vi "Update Sampling Rate.vi"(8 "error in (no error)":errorcluster, 10 "Timing Parameter":T1={"rate"=1000.0, "samples per channel"=1000, "sample mode"=10123} {"sample mode" items=["Finite Samples"=10178, "Continuous Samples"=10123, "Hardware Timed Single Point"=12522]; "rate" format="%0.2f"}, 11 "Abstract in":refnum<class "Abstract.lvclass">) -> (0 "error out":errorcluster, 3 "Abstract out":refnum<class "Abstract.lvclass">)   [LabVIEW 2016, in "DAQ Hardware.lvlib" / "Abstract.lvclass"]
uses:
  Abstract.lvclass
  Timing AI DAQ Setting.ctl
  DAQ Hardware.lvlib
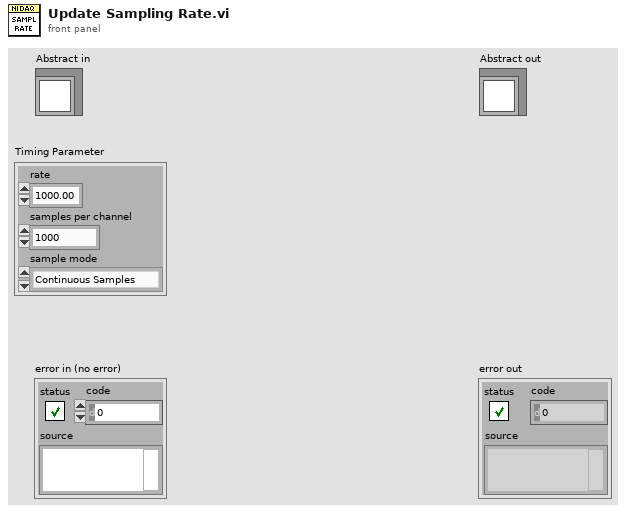
[diagram p1: front panel]
types:
  T1 = typedef "DAQ Hardware.lvlib/Timing AI DAQ Setting.ctl" = cluster{"rate":dbl, "samples per channel":i32, "sample mode":i32}
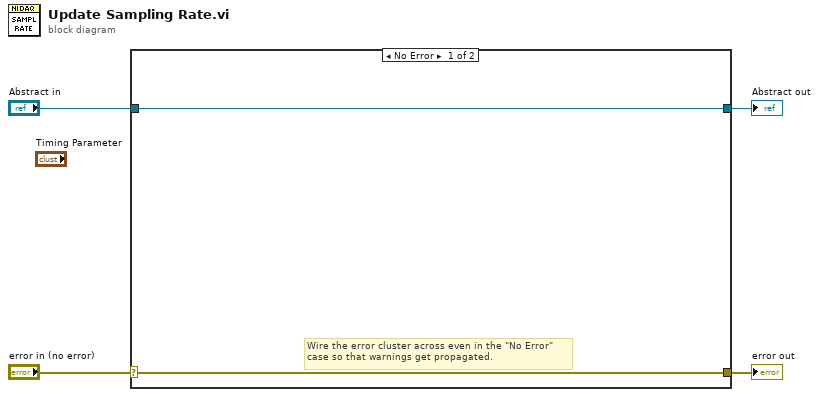
[diagram p0: block diagram]
diagram:
  n1 = case shown="No Error" "error in (no error)" {
    selector: "error in (no error)" -> [w5 w8]
    tunnel: [w5 w8] -> w3
    tunnel: [w6 w7] -> w1
    tunnel: "Abstract in" -> [w6 w7]
    frame No Error {
      # "Wire the error cluster across even in the \"No Error\"\ncase so that warnings get propagated."
    }
    frame Error {
    }
  }
  "error out" <- w3
  "Abstract out" <- w1
